vi "sub_read data.vi"(0 "Omega task":refnum<k24>[](array[refnum]), 5 "Omega error":errorcluster[](array[cluster]), 9 "Sensor task":refnum<k21>, 11 "Sensor error":errorcluster) -> (4 "Sensor Data":dbl[](array[numeric]), 6 "Sensor task out":refnum<k21>, 8 "Sensor error out":errorcluster, 10 "Omega task out":refnum<k24>[](array[refnum]), 13 "All initialized?":bool, 15 "Omega error out":errorcluster[](array[cluster]))   [LabVIEW 2020]
uses:
  C:/Program Files (x86)/National Instruments/LabVIEW 2020/vi.lib/ULx/ULx_LV.dll
  <vilib>/DAQmx/read.llb/DAQmx Read (Analog 1D DBL NChan 1Samp).vi
  <vilib>/DAQmx/miscellaneous.llb/DAQmx Fill In Error Info.vi
  <vilib>/ULx/Read.llb/ULx Read (Analog 1D DBL NChan 1Samp).vi
  globalvariables.vi
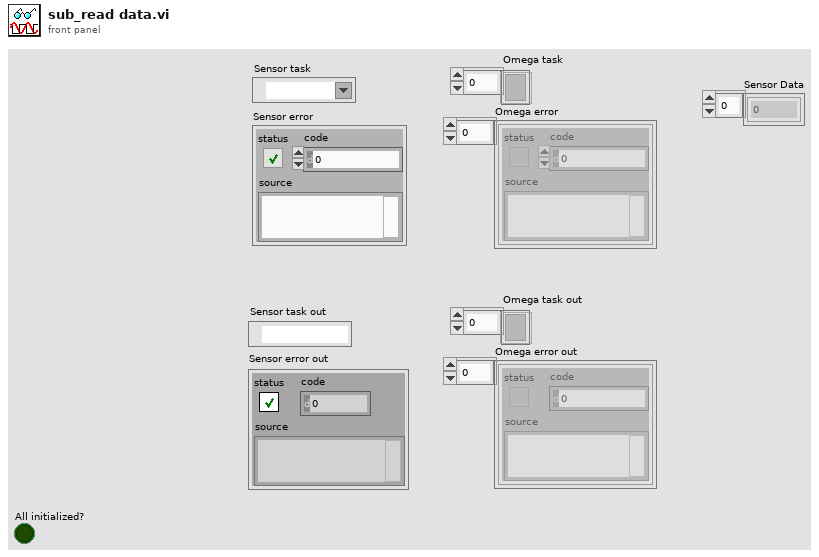
[diagram p1: front panel]
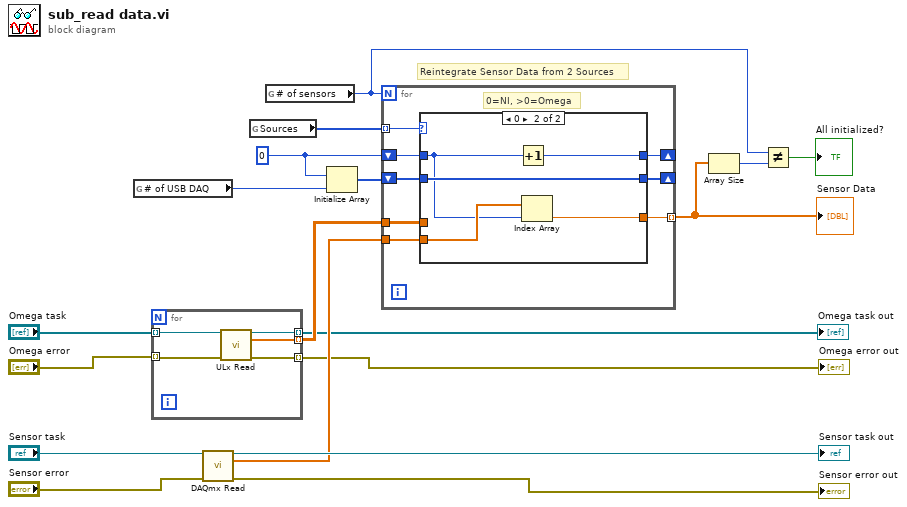
[diagram p0: block diagram]
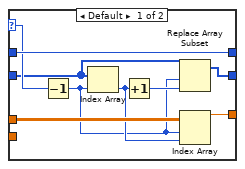
[diagram p2: hidden frame]
diagram:
  w6 = 0
  # "Reintegrate Sensor Data from 2 Sources"
  n1 = global read "globalvariables.vi" "# of USB DAQ"() -> (w5:i32)
  n2 = for {
    tunnel: [w23] -> w11 mode=indexing
    tunnel: "Omega error" -> [w22] mode=indexing
    tunnel: "Omega task" -> [w21] mode=indexing
    tunnel: [w20] -> w8 mode=indexing
    tunnel: [w19] -> w7 mode=indexing
    n3 = call-poly <vilib>:"ULx Read.vi"("task in"=w21, "error in"=w22) -> ("task out"=w20:refnum<k24>, "data"=w23:dbl[], "error out"=w19:errorcluster)  [unwired: 11 in]
  }
  "Omega task out" <- w8
  "Omega error out" <- w7
  n4 = call-poly <vilib>:"DAQmx Read.vi"("task/channels in"="Sensor task", "error in"="Sensor error") -> ("task out"=→"Sensor task out":refnum<k21>, "data"=w12:dbl[], "error out"=→"Sensor error out":errorcluster)  [unwired: 11 in]
  n5 = global read "globalvariables.vi" "Sources"() -> (w3:i32[])
  n6 = global read "globalvariables.vi" "# of sensors"() -> (w13:i32)
  n7 = Initialize Array(w6, w5) -> (w4:i32[])
  n8 = for {
    N: w13 -> [_]
    tunnel: w3 -> [w31] mode=indexing
    tunnel: w12 -> [w30]
    shift-right: [w26] -> _
    shift-left: w6 -> [w27]
    shift-right: [w28] -> _
    shift-left: w4 -> [w29]
    tunnel: [w25] -> w16 mode=indexing
    tunnel: w11 -> [w24]
    # "0=NI, >0=Omega"
    n9 = case shown="0" w31 {
      selector: w31 -> [w37 _]
      tunnel: w30 -> [_ w45]
      tunnel: w29 -> [w36 w44]
      tunnel: [w34 w44] -> w28
      tunnel: w27 -> [w40 w42]
      tunnel: [w40 w41] -> w26
      tunnel: [w39 w43] -> w25
      tunnel: w24 -> [w38 _]
      frame Default {
        n10 = Decrement(x=w37) -> (x-1=w32:i32)
        n11 = Index Array(array=w36, index=w32) -> (element=w33:i32)
        n12 = Increment(x=w33) -> (x+1=w35:i32)
        n13 = Replace Array Subset(array=w36, new element=w35, index=w32) -> (w34:i32[])
        n14 = Index Array(array=w38, index (row)=w32, index (col)=w33) -> (element=w39:dbl)
      }
      frame 0 {
        n15 = Increment(x=w42) -> (x+1=w41:i32)
        n16 = Index Array(array=w45, index=w42) -> (element=w43:dbl)
      }
    }
  }
  "Sensor Data" <- w16
  n17 = Array Size(array=w16) -> (size(s)=w15:i32)
  n18 = Not Equal?(x=w13, y=w15) -> (x != y?=→"All initialized?":bool)
